vi "Day 5 task 2.vi"() -> ()   [LabVIEW 2022 SP3]
panel:
  in  "stop":bool
  out "Location":i32
  out "Seed":u64
  out "min value":u64
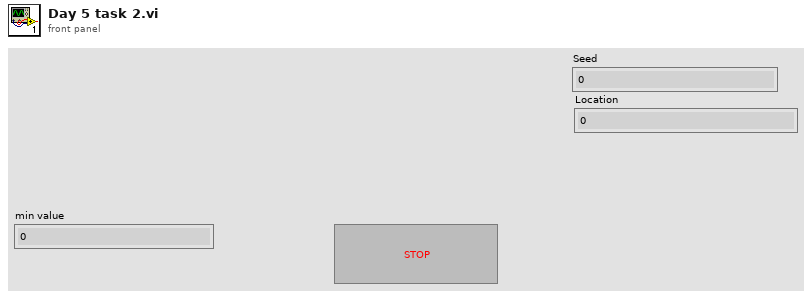
[diagram p1: front panel]
types:
  T1 = map{cluster{"Start":u64, "End":u64}, cluster{"Start":u64, "End":u64}}
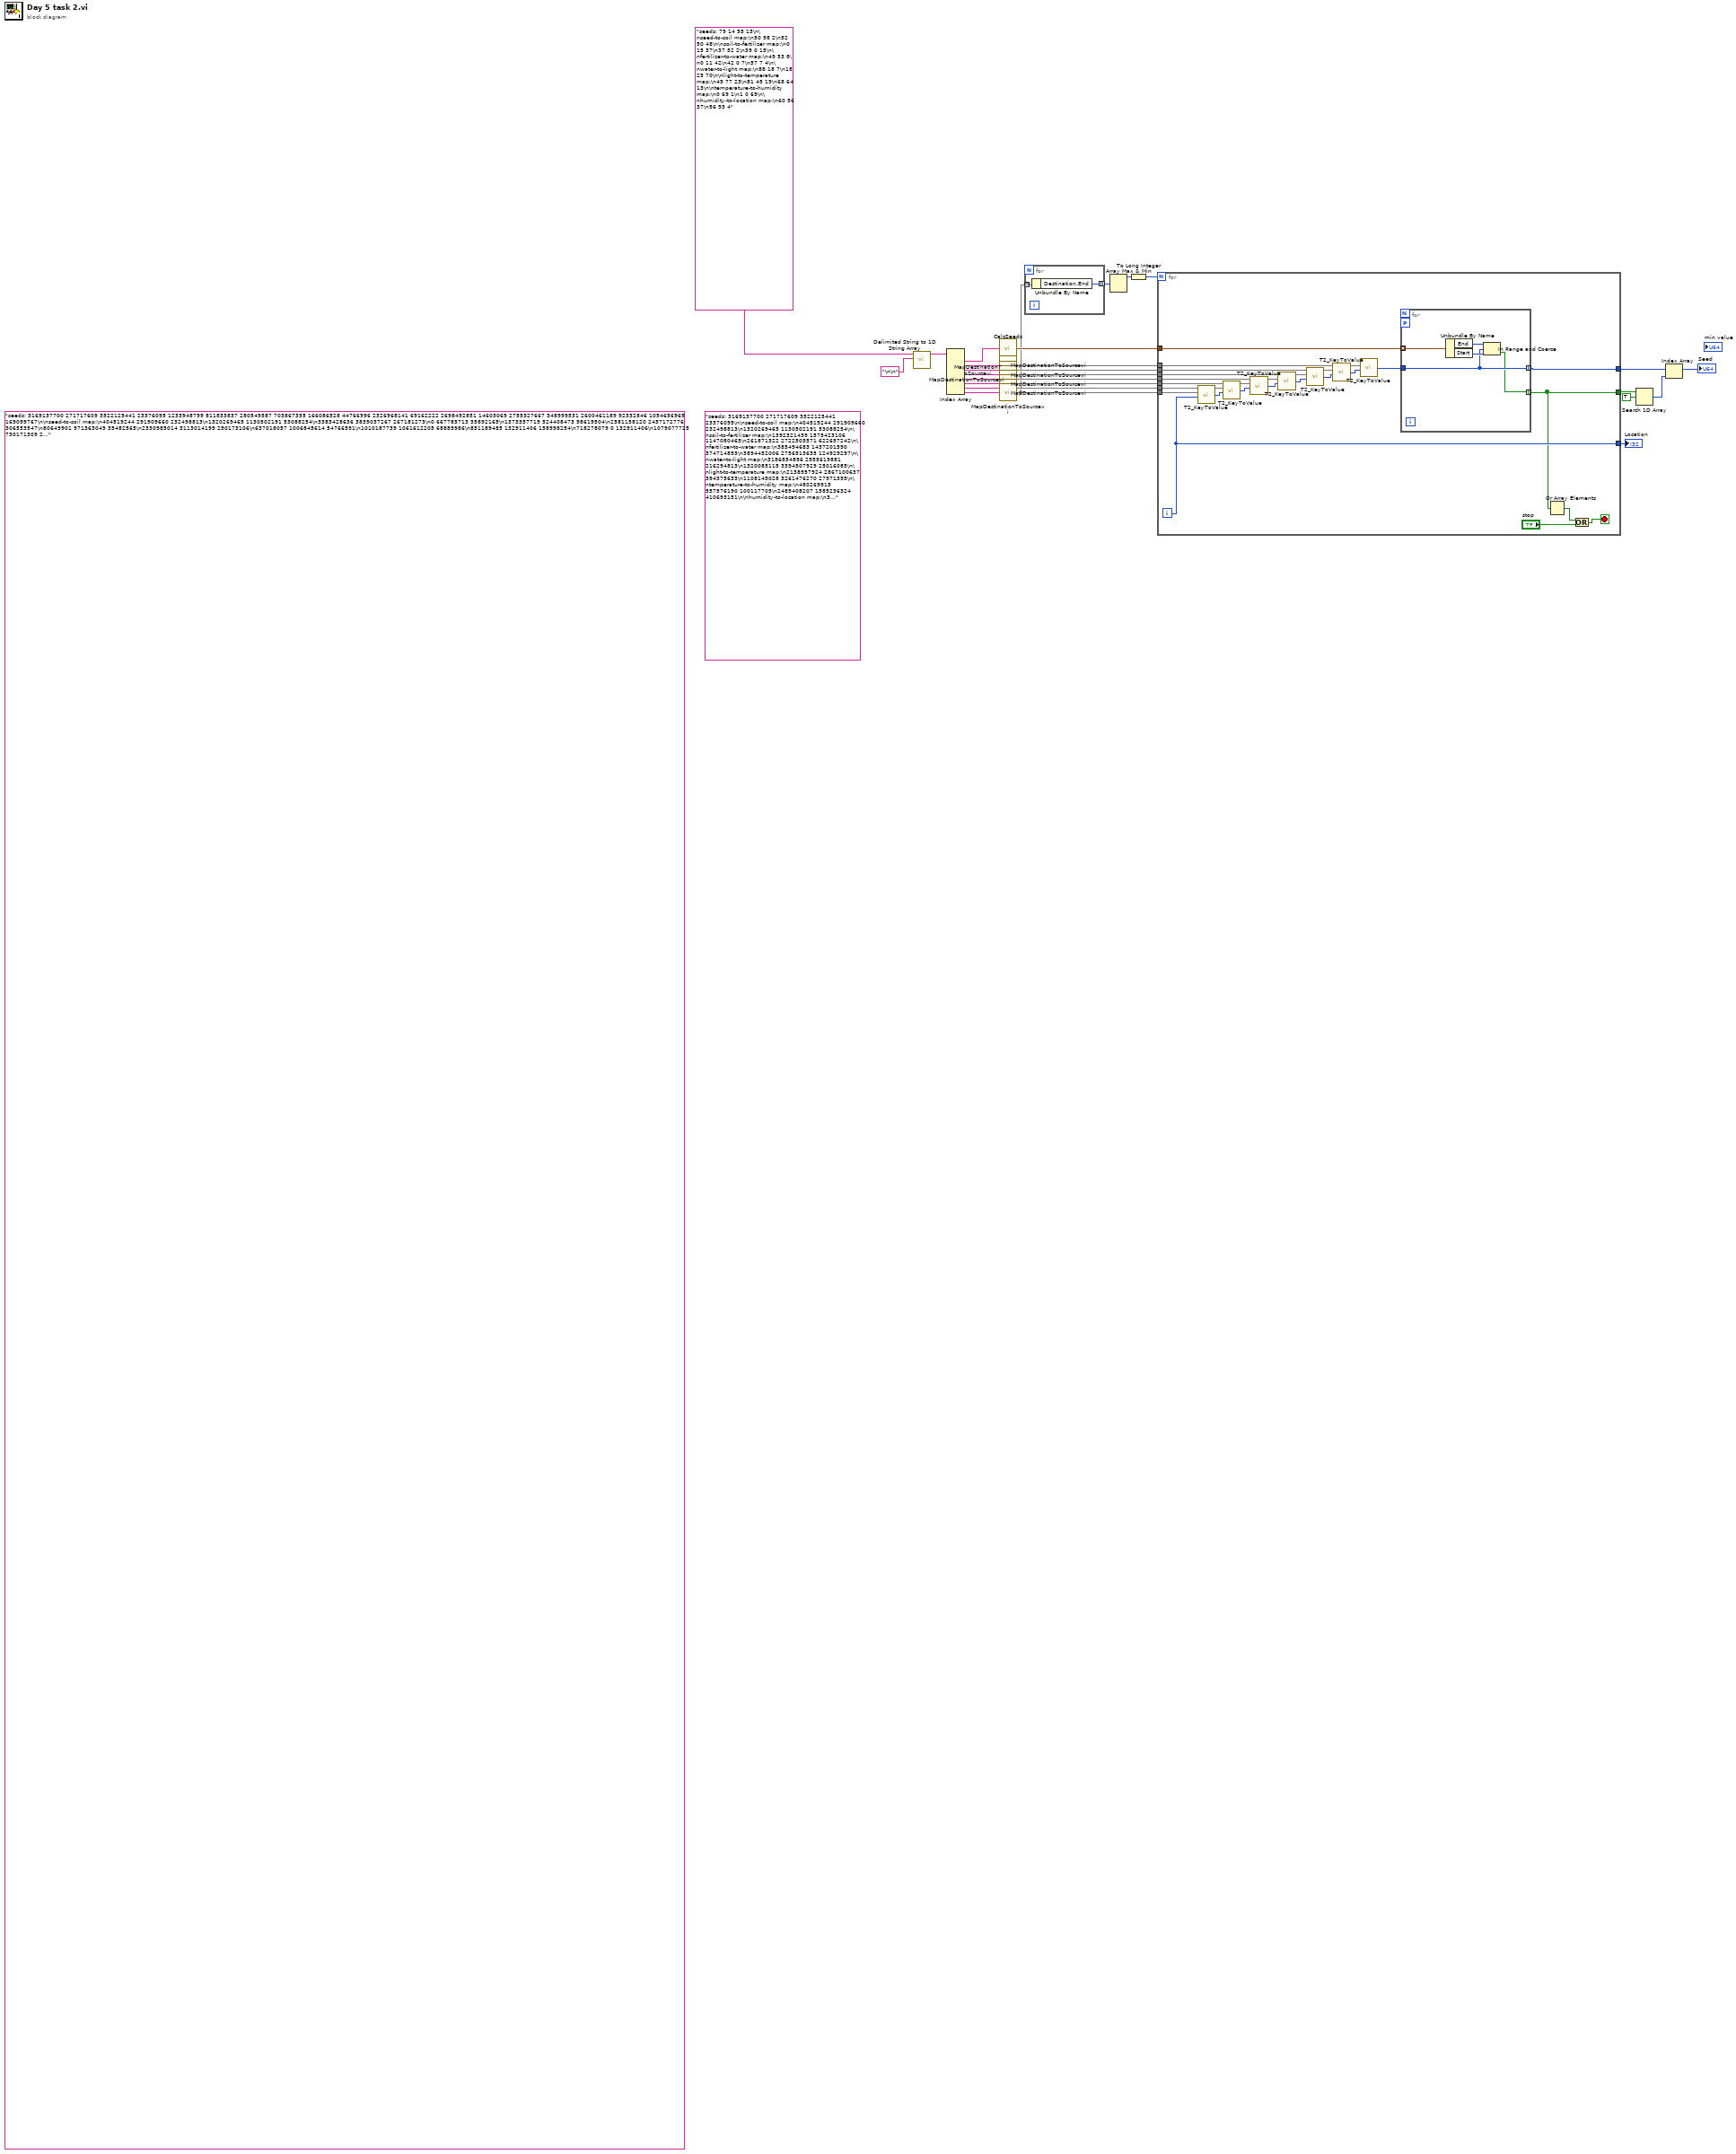
[diagram p0: block diagram]
diagram:
  (unwired) "seeds: 3169137700 271717609 3522125441 23376095 1233948799 811833837 280549587 703867355 166086528 44766996 2326968141 69162222 2698492851 14603069 2755327667 348999531 2600461189 92332846 1054656969 169099767\n\nseed-to-soil map:\n404519244 291909660 232498813\n1320269465 1130502191 53088254\n3383428636 3839037267 267181273\n0 667785713 35892165\n1373357719 524408473 98619504\n2581158120 2457172776 306553547\n80649901 971363049 35482565\n2330985014 3113014199 250173106\n637018057 1006845614 54766591\n1010187739 1061612205 68889986\n851189485 132911406 158998254\n718278079 0 132911406\n1079077725 730171309 241191740\n2887711667 2392582028 64590748\n3321831622 2330985014 61597014\n3650609909 4106218540 188748756\n2952302415 3363187305 20241331\n368073252 1183590445 36445992\n3839358665 3383428636 455608631\n35892165 623027977 44757736\n2972543746 2763726323 349287876\n691784648 703677878 26493431\n116132466 1220036437 251940786\n\nsoil-to-fertilizer map:\n1392321439 1575423106 1147080465\n261871322 2722503571 622657242\n884528564 768981668 507792875\n3152000765 0 514557996\n2539401904 3607032135 247383303\n2786785207 3854415438 110791886\n2897577093 514557996 254423672\n3666558761 1276774543 298648563\n0 3345160813 261871322\n\nfertilizer-to-water map:\n385494683 1437201590 374714893\n3894452006 2756513635 124929297\n1389571244 1299917000 137284590\n3267934068 2881442932 9378230\n4140946106 2602492445 154021190\n760209576 585965354 629361668\n1948388381 1832044460 70164711\n170741915 176668131 214752768\n3570093835 2531499423 70993022\n2647843344 3421511423 399466167\n1832044460 3124261283 116343921\n3458218517 2890821162 111875318\n1721400289 1215327022 84589978\n1526855834 391420899 194544455\n4019381303 3002696480 121564803\n3641086857 4041602147 253365149\n2018553092 1902209171 629290252\n3047309511 3820977590 220624557\n1805990267 170741915 5926216\n3277312298 3240605204 180906219\n\nwater-to-light map:\n3186854896 2955619881 216294813\n1320085115 3394507929 25016085\n1300936985 1818141535 19148130\n3620767971 560782805 39686383\n2121550779 2395592136 95582251\n3594740149 4260270958 26027822\n1138228493 3171914694 34259798\n823736132 600469188 55727065\n3049715340 2803112532 137139556\n0 461804882 98977923\n2217133030 1416346841 282474073\n1225320767 1742525317 75616218\n3481284141 3206174492 113456008\n1172488291 656196253 52832476\n1980983454 2662545207 140567325\n182051501 2121838778 15960124\n1788572787 256566375 2332800\n881662118 0 256566375\n3769058535 899106596 517240245\n157917514 3851650114 24133987\n564440564 1937530266 107354197\n2527210819 4090588051 169682907\n1790905587 709028729 190077867\n2499607103 3824046398 27603716\n1585667080 258899175 202905707\n671794761 3419524014 51700770\n3403149709 2491174387 62766639\n228474519 2044884463 76954315\n3660454354 2553941026 108604181\n305428834 2137798902 257793234\n879463197 3875784101 2198921\n2696893726 3471224784 352821614\n1345101200 3319630500 74877429\n98977923 4031648460 58939591\n1541962677 1698820914 43704403\n3465916348 2940252088 15367793\n1419978629 3909664412 121984048\n723495531 1837289665 100240601\n563222068 3908445916 1218496\n198011625 3877983022 30462894\n\nlight-to-temperature map:\n2138957924 2867100637 394375633\n1108145028 3261476270 27971395\n2732973434 712143665 259385506\n642453123 1589178663 51870752\n316125718 164593015 67732689\n0 145842404 18750611\n1861017768 2758655274 29719920\n2130609825 2858752538 8348099\n828190830 2187066385 73864838\n18750611 0 126160197\n144910808 376698573 26842041\n383858407 126160197 19682207\n2533333557 3337386080 199639877\n1507332395 1950588856 215367909\n3619117542 3537025957 51848058\n1740303803 1763491162 21707209\n3793407347 4140330531 154636765\n477829952 3588874015 164623171\n1722700304 1432603163 17603499\n1890737688 493381148 218762517\n4255326359 1549537726 39640937\n1408001331 1450206662 99331064\n2992358940 2260931223 497724051\n429891537 3289447665 47938415\n3670965600 1641049415 122441747\n171752849 232325704 144372869\n3504169105 3753497186 114948437\n2109500205 2165956765 21109620\n4113434597 1290711401 141891762\n3490082991 1070535927 14086114\n1136116423 3868445623 271884908\n757813486 2788375194 70377344\n3948044112 1785198371 165390485\n694323875 429891537 63489611\n1762011012 971529171 99006756\n902055668 1084622041 206089360\n\ntemperature-to-humidity map:\n480269915 557576190 100117705\n2489408207 1585236324 410693151\n2900101358 422045351 135530839\n666327594 779006907 28457451\n1945409298 807464358 543998909\n96132998 2440771002 3096292\n1295929224 2746460169 2283706\n1298212930 2022055443 99310345\n3547441134 3503466915 344864128\n1659646920 325230280 96815071\n4125576596 3928494543 169390700\n3035632197 1351463267 233773057\n1397523275 2592671813 109157546\n1032938960 2748743875 109076238\n1756461991 2276586008 92935317\n3968917823 4097885243 156658773\n595077917 2369521325 71249677\n1593864657 3027700045 65782263\n850005265 657693895 121313012\n1506680821 2505487977 87183836\n1186646008 0 109283216\n1849397308 3389340328 96011990\n3496945571 4254544016 40423280\n3898826606 3858403326 70091217\n99229290 3189615306 199725022\n468834244 1995929475 11435671\n3269405254 109283216 215947064\n580387620 2007365146 14690297\n0 3093482308 96132998\n971318277 2443867294 61620683\n3892305262 3496945571 6521344\n298954312 2857820113 169879932\n1142015198 2701829359 44630810\n694785045 2121365788 155220220\n3537368851 3848331043 10072283\n\nhumidity-to-location map:\n3490144003 1623866227 218040905\n1709610578 1620839197 3027030\n105449249 586389428 113279526\n1899604338 2167886292 348178199\n1712637608 2678624215 186966730\n218728775 0 245776251\n2472992580 923734334 143670388\n2616662968 3670169885 15297294\n2247782537 1395629154 225210043\n0 480940179 105449249\n4113852846 3959729057 159909096\n3322784653 1067404722 167359350\n923734334 4119638153 175329143\n1534964496 2516064491 162559724\n2631960262 3496028440 140849733\n2862695906 1234764072 97988355\n1697524220 3636878173 12086358\n2985646048 1332752427 62876727\n1099063477 2970241510 435901019\n4009202281 2865590945 104650565\n2960684261 2142924505 24961787\n2772809995 3406142529 89885911\n4273761942 3648964531 21205354\n3708184908 1841907132 301017373\n464505026 245776251 235163928\n3048522775 3685467179 274261878"
  (unwired) "seeds: 3169137700 271717609 3522125441 23376095\n\nseed-to-soil map:\n404519244 291909660 232498813\n1320269465 1130502191 53088254\n\nsoil-to-fertilizer map:\n1392321439 1575423106 1147080465\n261871322 2722503571 622657242\n\nfertilizer-to-water map:\n385494683 1437201590 374714893\n3894452006 2756513635 124929297\n\nwater-to-light map:\n3186854896 2955619881 216294813\n1320085115 3394507929 25016085\n\nlight-to-temperature map:\n2138957924 2867100637 394375633\n1108145028 3261476270 27971395\n\ntemperature-to-humidity map:\n480269915 557576190 100117705\n2489408207 1585236324 410693151\n\nhumidity-to-location map:\n3490144003 1623866227 218040905\n1709610578 1620839197 3027030"
  n1 = call <vilib>:"Delimited String to 1D String Array.vi"("delimiter"="\n\n", "delimited string"="seeds: 79 14 55 13\n\nseed-to-soil map:\n50 98 2\n52 50 48\n\nsoil-to-fertilizer map:\n0 15 37\n37 52 2\n39 0 15\n\nfertilizer-to-water map:\n49 53 8\n0 11 42\n42 0 7\n57 7 4\n\nwater-to-light map:\n88 18 7\n18 25 70\n\nlight-to-temperature map:\n45 77 23\n81 45 19\n68 64 13\n\ntemperature-to-humidity map:\n0 69 1\n1 0 69\n\nhumidity-to-location map:\n60 56 37\n56 93 4") -> ("string array"=w27:string[])  [unwired: 9 in]
  n2 = Index Array(array=w27) -> (element #1=w13:string, element #2=w26:string, element #3=w25:string, element #4=w24:string, element #5=w23:string, element #6=w22:string, element #7=w21:string, element #8=w20:string)  [unwired: 8 in]
  n3 = call "CalcSeeds.vi"("String"=w13) -> ("Seeds"=w12:cluster{"Start":u64, "End":u64}[])  [unwired: 6 in]
  n4 = call "MapDestinationToSourcevi.vi"("String"=w26) -> ("Dest > Source"=w14:T1)  [unwired: 6 in]
  n5 = call "MapDestinationToSourcevi.vi"("String"=w25) -> ("Dest > Source"=w15:T1)  [unwired: 6 in]
  n6 = call "MapDestinationToSourcevi.vi"("String"=w24) -> ("Dest > Source"=w16:T1)  [unwired: 6 in]
  n7 = call "MapDestinationToSourcevi.vi"("String"=w23) -> ("Dest > Source"=w17:T1)  [unwired: 6 in]
  n8 = call "MapDestinationToSourcevi.vi"("String"=w22) -> ("Dest > Source"=w18:T1)  [unwired: 6 in]
  n9 = call "MapDestinationToSourcevi.vi"("String"=w21) -> ("Dest > Source"=w19:T1)  [unwired: 6 in]
  n10 = call "MapDestinationToSourcevi.vi"("String"=w20) -> ("Dest > Source"=w5:T1)  [unwired: 6 in]
  n11 = for {
    tunnel: w5 -> [w30] mode=indexing
    tunnel: [w29] -> w4 mode=indexing
    n12 = Unbundle By Name(w30) -> ("Destination.End"=w29:u64)
  }
  n13 = Array Max & Min(array=w4) -> (max value=w3:u64)  [unwired: 3 out]
  n14 = To Long Integer(number=w3) -> (32bit integer=w2:i32)
  n15 = for {
    N: w2 -> [_]
    tunnel: w14 -> [w51]
    tunnel: w15 -> [w50]
    tunnel: w16 -> [w49]
    tunnel: w17 -> [w48]
    tunnel: w18 -> [w47]
    tunnel: w19 -> [w46]
    tunnel: w5 -> [w45]
    tunnel: w12 -> [w38]
    tunnel: [w36] -> w11
    tunnel: [w35] -> w10
    tunnel: [w34] -> w9
    i -> [w35]
    stop <- w33 stop-if-true
    n16 = call "T2_KeyToValue.vi"("Key"=w35, "Source > Dest"=w45) -> ("Value"=w44:u64)  [unwired: 4 in]
    n17 = call "T2_KeyToValue.vi"("Key"=w44, "Source > Dest"=w46) -> ("Value"=w43:u64)  [unwired: 4 in]
    n18 = call "T2_KeyToValue.vi"("Key"=w43, "Source > Dest"=w47) -> ("Value"=w42:u64)  [unwired: 4 in]
    n19 = call "T2_KeyToValue.vi"("Key"=w42, "Source > Dest"=w48) -> ("Value"=w41:u64)  [unwired: 4 in]
    n20 = call "T2_KeyToValue.vi"("Key"=w41, "Source > Dest"=w49) -> ("Value"=w40:u64)  [unwired: 4 in]
    n21 = call "T2_KeyToValue.vi"("Key"=w40, "Source > Dest"=w50) -> ("Value"=w39:u64)  [unwired: 4 in]
    n22 = call "T2_KeyToValue.vi"("Key"=w39, "Source > Dest"=w51) -> ("Value"=w37:u64)  [unwired: 4 in]
    n23 = for {
      tunnel: w38 -> [w56] mode=indexing
      tunnel: w37 -> [w53]
      tunnel: [w53] -> w36 mode=indexing
      tunnel: [w52] -> w34 mode=indexing
      workers-P: _ -> [_]
      n24 = Unbundle By Name(w56) -> ("End"=w54:u64, "Start"=w55:u64)
      n25 = In Range and Coerce(upper limit=w54, x=w53, lower limit=w55) -> (In Range?=w52:bool)  [unwired: 1 out]
    }
    n26 = Or Array Elements(Boolean array=w34) -> (logical OR=w32:bool)
    n27 = Or(x=w32, y="stop") -> (x .or. y?=w33:bool)
  }
  "Location" <- w10
  n28 = Search 1D Array(1D array=w9, element=TRUE) -> (index of element=w6:i32)  [unwired: 1 in]
  n29 = Index Array(array=w11, index=w6) -> (element=→"Seed":u64)
